vi "Obtain Real Class.vi"(8 "error in (no error)":errorcluster, 11 "Shape":refnum<data-value>) -> (0 "error out":errorcluster, 3 "Inner Shape":refnum<data-value>)   [LabVIEW 2017, in "LV Image Editor Framework.lvlib" / "Selection.lvclass"]
uses:
  <vilib>/LIEF/Forms/Selection/Selection.lvclass
  <vilib>/LIEF/Forms/Shape/Shape.lvclass
  <vilib>/LIEF/Forms/Selection/Selection.lvclass/Selection.ctl
  <vilib>/LIEF/Forms/Selection/Read Selected Shape.vi
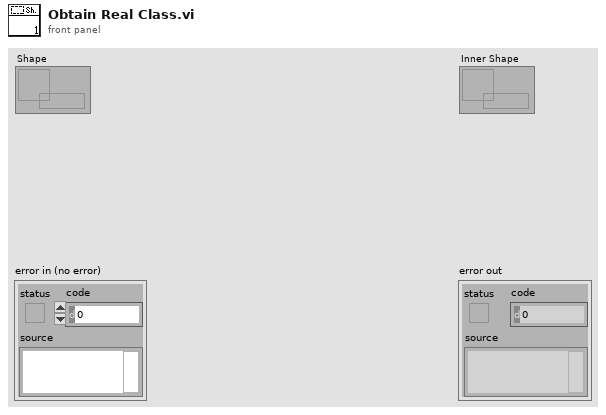
[diagram p1: front panel]
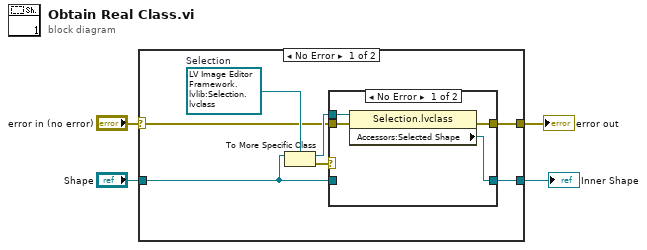
[diagram p0: block diagram]
diagram:
  n1 = case shown="No Error" "error in (no error)" {
    selector: "error in (no error)" -> [w6 w19]
    tunnel: [w5 w19] -> w3
    tunnel: "Shape" -> [w9 w18]
    tunnel: [w7 w18] -> w1
    frame No Error {
      w11 = refnum<data-value> refnum  # Selection
      n2 = To More Specific Class(target class=w11, reference=w9) -> (specific class reference=w10:refnum<data-value>, error out=w8:errorcluster)  [unwired: 1 in]
      n3 = case shown="No Error" w8 {
        tunnel: w10 -> [w15 _]
        tunnel: w9 -> [_ w17]
        tunnel: [w14 w17] -> w7
        tunnel: w6 -> [w13 w16]
        tunnel: [w12 w16] -> w5
        frame No Error {
          n4 = property class="Selection.lvclass"(reference=w15, error in=w13) -> (error out=w12:errorcluster, "Accessors:Selected Shape"=w14:refnum<data-value>)  [unwired: 1 out]
        }
        frame Error {
        }
      }
    }
    frame Error {
    }
  }
  "error out" <- w3
  "Inner Shape" <- w1
